vi "ChannelType_Anything.vi"(9 "error in":errorcluster, 11 "Anything in":refnum<class "Anything.lvclass">) -> (1 "error out":errorcluster, 2 "ChannelType":refnum<class "Anything.lvclass">, 3 "Anything out":refnum<class "Anything.lvclass">)   [LabVIEW 2020, in "OpenLvVision_OpenCv.lvlib"]
uses:
  OpenLvVision_OpenCv.lvlib
  Anything.lvclass
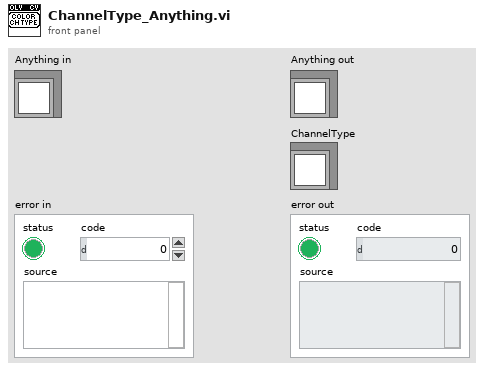
[diagram p1: front panel]
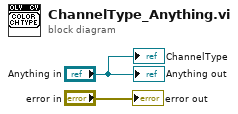
[diagram p0: block diagram]
diagram:
  "Anything out" <- "Anything in"
  "error out" <- "error in"
  "ChannelType" <- "Anything in"
